vi "WSVCAP SHL Host LL Initialize Top Level Controls Manager.vi"(1 "FPGA VI Reference (Init Only)":T2, 11 "error in (no error)":errorcluster, 12 "Simulate FPGA (Init Only)":bool=TRUE, 14 "FPGA":T1) -> (15 "error out":errorcluster)   [LabVIEW 2017]
uses:
  Type Defs/WSVCAP SHL FPGA Ref.ctl
  Type Defs/WSVCAP SHL FPGA Enum.ctl
  Type Defs/WSVCAP SHL Top Level Control Operation Enum.ctl
  Type Defs/WSVCAP SHL Gatekeeper Operation Enum.ctl
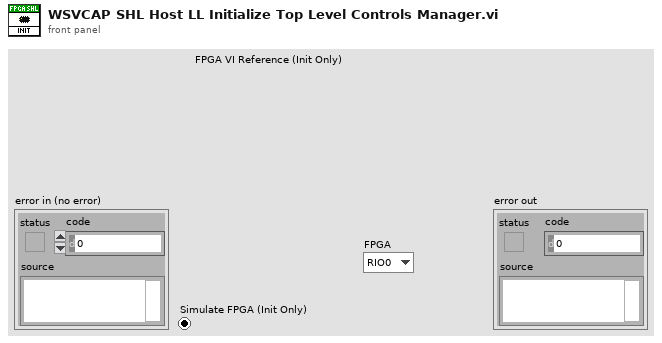
[diagram p1: front panel]
types:
  T1 = typedef "WSVCAP SHL FPGA Enum.ctl" = enum16{"RIO0", "RIO1"}
  T2 = typedef "WSVCAP SHL FPGA Ref.ctl" = refnum<k20>
  T3 = typedef "WSVCAP SHL Gatekeeper Operation Enum.ctl" = enum16{"Initialize", "Lock", "Unlock", "Close"}
  T4 = typedef "WSVCAP SHL Top Level Control Operation Enum.ctl" = enum16{"Initialize", "Set Control", "Read Control", "Close"}
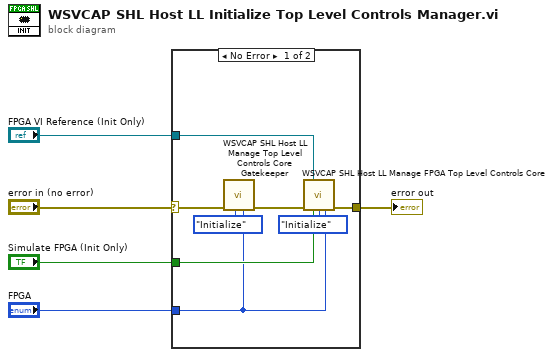
[diagram p0: block diagram]
diagram:
  n1 = case shown="No Error" "error in (no error)" {
    selector: "error in (no error)" -> [w8 w14]
    tunnel: [w12 w14] -> w5
    tunnel: "Simulate FPGA (Init Only)" -> [w11 _]
    tunnel: "FPGA" -> [w6 _]
    tunnel: "FPGA VI Reference (Init Only)" -> [w10 _]
    frame No Error {
      n2 = call "WSVCAP SHL Host LL Manage Top Level Controls Core Gatekeeper.vi"("FPGA"=w6, "Operation"=WSVCAP_SHL_Gatekeeper_Operation_Enum."Initialize", "error in (no error)"=w8) -> ("error out"=w7:errorcluster)  [unwired: 8 in]
      n3 = call "WSVCAP SHL Host LL Manage FPGA Top Level Controls Core.vi"("FPGA VI Reference (Init Only)"=w10, "error in (no error)"=w7, "Simulate FPGA (Init Only)"=w11, "Operation"=WSVCAP_SHL_Top_Level_Control_Operation_Enum."Initialize", "FPGA"=w6) -> ("error out"=w12:errorcluster)  [unwired: 9 in, 1 out]
    }
    frame Error {
    }
  }
  "error out" <- w5
